vi "Add Files to Project.vi"   [LabVIEW 2023]
doc: "This VI adds all VIs listed in the \"Top Level VIs to Add to Project\" array to a new project, and then adds all the directories (and their files) listed in the \"Top Level Folders to Add to Project\" array to the project."
panel:
  # "Overview: Demonstrates the use of VI Server to programmatically manipulate a LabVIEW Project.\nInstructions:\nRun the VI. A new LabVIEW Project is created and populated programmatically.  See the block diagram for more information."
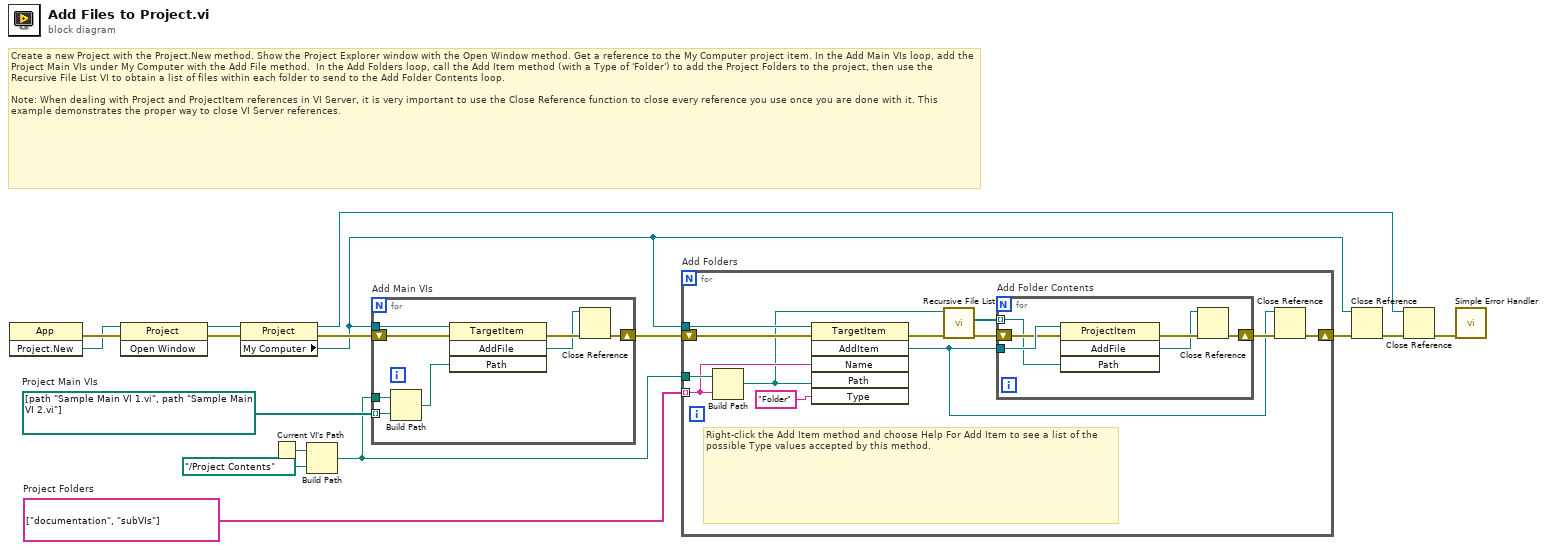
[diagram p0: block diagram]
diagram:
  w12 = string[] ["documentation", "subVIs"]  # Project Folders
  w13 = path[] [path "Sample Main VI 1.vi", path "Sample Main VI 2.vi"]  # Project Main VIs
  # "Create a new Project with the Project.New method. Show the Project Explorer window with the Open Window method. Get a reference to the My Computer project item. In the Add Main VIs loop, add the Project Main VIs under My Computer with the Add File method.  In the Add Folders loop, call the Add Item method (with a Type of 'Folder') to add the Project Folders to the project, then use the Recursive File List VI to obtain a list of files within each folder to send to the Add Folder Contents loop.\n\nNote: When dealing with Project and ProjectItem references in VI Server, it is very important to use the Close Reference function to close every reference you use once you are done with it. This example demonstrates the proper way to close VI Server references."
  n1 = invoke class="App" method="Project.New"() -> (error out=w16:errorcluster, "Project:New"=w9:refnum<vi>)  [unwired: 3 in, 1 out]
  n2 = invoke class="Project" method="Open Window"(reference=w9, error in=w16) -> (reference out=w15:refnum<vi>, error out=w14:errorcluster)  [unwired: 1 in, 1 out]
  n3 = property class="Project"(reference=w15, error in=w14) -> (reference out=w4:refnum<vi>, error out=w8:errorcluster, "My Computer"=w5:refnum<vi>)
  n4 = Current VI's Path() -> (path=w2:path)
  n5 = Build Path(base path=w2, name or relative path=path "../Project Contents") -> (appended path=w3:path)
  n6 = for "Add Main VIs" {
    tunnel: w13 -> [w19] mode=indexing
    tunnel: w3 -> [w23]
    shift-right: [w18] -> w11
    shift-left: w8 -> [w21]
    tunnel: w5 -> [w24]
    n7 = Build Path(base path=w23, name or relative path=w19) -> (appended path=w22:path)
    n8 = invoke class="TargetItem" method="AddFile"(reference=w24, error in=w21, "Path"=w22) -> (error out=w20:errorcluster, "AddFile"=w17:refnum<vi>)  [unwired: 1 in, 2 out]
    n9 = Close Reference(reference=w17, error in (no error)=w20) -> (error out=w18:errorcluster)
  }
  n10 = for "Add Folders" {
    tunnel: w12 -> [w34] mode=indexing
    tunnel: w3 -> [w36]
    tunnel: w5 -> [w35]
    shift-right: [w26] -> w10
    shift-left: w11 -> [w33]
    # "Right-click the Add Item method and choose Help For Add Item to see a list of the possible Type values accepted by this method."
    n11 = Build Path(base path=w36, name or relative path=w34) -> (appended path=w27:path)
    n12 = invoke class="TargetItem" method="AddItem"(reference=w35, error in=w33, "Name"=w34, "Path"=w27, "Type"="Folder") -> (error out=w31:errorcluster, "AddItem"=w25:refnum<vi>)  [unwired: 1 in, 4 out]
    n13 = call <vilib>:"Recursive File List.vi"("error in (no error)"=w31, "Folder Path"=w27) -> ("error out"=w30:errorcluster, "All Files in Dir"=w29:path[])  [unwired: 5 in, 3 out]
    n14 = for "Add Folder Contents" {
      tunnel: w25 -> [w42]
      shift-right: [w38] -> w32
      shift-left: w30 -> [w41]
      tunnel: w29 -> [w39] mode=indexing
      n15 = invoke class="ProjectItem" method="AddFile"(reference=w42, error in=w41, "Path"=w39) -> (error out=w40:errorcluster, "AddFile"=w37:refnum<vi>)  [unwired: 1 in, 2 out]
      n16 = Close Reference(reference=w37, error in (no error)=w40) -> (error out=w38:errorcluster)
    }
    n17 = Close Reference(reference=w25, error in (no error)=w32) -> (error out=w26:errorcluster)
  }
  n18 = Close Reference(reference=w5, error in (no error)=w10) -> (error out=w7:errorcluster)
  n19 = Close Reference(reference=w4, error in (no error)=w7) -> (error out=w6:errorcluster)
  n20 = call <vilib>:"Simple Error Handler.vi"("error in (no error)"=w6) -> ()  [unwired: 1 in, 8 out]
